vi "Sync.vi"(8 "Error In":errorcluster, 11 "SFTP File In":refnum<class "SFTP File.lvclass">) -> (0 "Error Out":errorcluster, 3 "SFTP File Out":refnum<class "SFTP File.lvclass">)   [LabVIEW 2018, in "Toolkit.lvlib" / "SFTP File.lvclass"]
uses:
  SFTP File.lvclass
  SFTP File.lvclass/SFTP File.ctl
  SFTP/SFTP.lvclass/SFTP.ctl
  Toolkit.lvlib
  SFTP/SFTP.lvclass
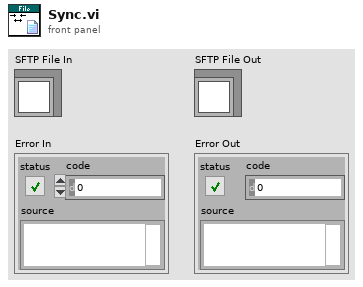
[diagram p1: front panel]
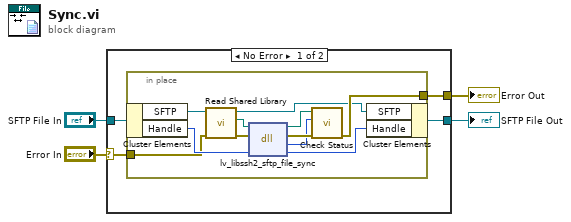
[diagram p0: block diagram]
diagram:
  n1 = case shown="No Error" "Error In" {
    selector: "Error In" -> [w7 w20]
    tunnel: "SFTP File In" -> [w8 w21]
    tunnel: [w6 w21] -> w1
    tunnel: [w5 w20] -> w2
    frame No Error {
      n2 = in-place {
        in-place-border: w7 -> [w18]
        in-place-border: [w13] -> w5
        n3 = in-place-cluster #1(w8) -> ("SFTP"=w11:refnum<class "SFTP.lvclass">, "Handle"=w19:u64)
        n4 = call "Read Shared Library.vi"("Error In"=w18, "SFTP In"=w11) -> ("Erorr Out"=w12:errorcluster, "lv-libssh2 Shared Library"=w9:path, "SFTP Out"=w10:refnum<class "SFTP.lvclass">)  [unwired: 7 in]
        n5 = dll-call lib="libssh2lv.*" fn="lv_libssh2_sftp_file_sync"(path in=w9, error in=w12, "handle"=w19) -> (path out=w15:path, error out=w16:errorcluster, "status"=w14:i32, "handle"=w17:u64)  [unwired: 1 in]
        n6 = call "Check Status.vi"("Error In"=w16, "Status"=w14, "lv-libssh2 Shared Library In"=w15) -> ("Error Out"=w13:errorcluster)  [unwired: 7 in, 1 out]
        n7 = in-place-cluster #1("SFTP"=w10, "Handle"=w17) -> (w6:refnum<class "SFTP File.lvclass">)
      }
    }
    frame Error {
    }
  }
  "Error Out" <- w2
  "SFTP File Out" <- w1
